vi "SetZControl.vi"(0 "Z Control Cluster":T1={"Input Signal"=0, "Min"=-inf, "Max"=-inf, "P"=-inf, "Setpoint a.u."=-inf, "Invert Polarity"=-2147483648, "I"=-inf} {"I" format="%#_g mHz"; "Invert Polarity" items=["[read only]"=-2147483648, "No"=0, "Yes"=1]; "Max" format="%#_g nm"; "Min" format="%#_g nm"; "Input Signal" items=["[read only]"=-2147483648, "ADC 1"=0, "ADC 2"=1, "ADC 3"=2, "ADC 4"=3, "ADC 5"=4, "ADC 6"=5, "HF 1 df"=8, "HF 1 Ampl"=13, "HF 1 Phase"=14, "LockIn Ampl"=16, "LockIn Phase"=17, "Counter"=23]}, 5 "error in":T4) -> (14 "Z Control Output":T1={"Input Signal"=0, "Min"=-inf, "Max"=-inf, "P"=-inf, "Setpoint a.u."=-inf, "Invert Polarity"=-2147483648, "I"=-inf} {"I" format="%#_g mHz"; "Invert Polarity" items=["[read only]"=-2147483648, "No"=0, "Yes"=1]; "Max" format="%#_g nm"; "Min" format="%#_g nm"; "Input Signal" items=["[read only]"=-2147483648, "ADC 1"=0, "ADC 2"=1, "ADC 3"=2, "ADC 4"=3, "ADC 5"=4, "ADC 6"=5, "HF 1 df"=8, "HF 1 Ampl"=13, "HF 1 Phase"=14, "LockIn Ampl"=16, "LockIn Phase"=17, "Counter"=23]}, 19 "error out":T4)   [LabVIEW 2016]
doc: "This VI prepares the z control by setting up all necessary parameters. Those are bundled in 'Z Control Cluster':\n\n- Actual Value (integer) [0-5 -- ADC1-6; 8 -- AFM df; 13 -- AFM Aosc; 14 -- AFM Phase; 16 -- LockIn Ampl; 17 -- LockIn Phase]\n- Min in nm (float) [0 to infinity]\n- Max in nm (float) [0 to infinity]\n- P (float) [0 to 100]\n- I in mHz (float) [without restraint]\n- Setpoint in mV, Hz or deg depending on the input \"Actual Value\". (float) [without restraint]\n- Invert Polarity (integer) [0 -- no; 1 -- yes]\n- Absolute (integer) [0 -- off; 1 -- on]\nBy passing -Inf (float) or -2147483648 (integer) as input values, the corresponding parameter(s) will be read out."
uses:
  Controls/Error_Out.ctl
  Controls/Z-Control_Parameters.ctl
  Controls/Actual-Value_Selection.ctl
  Controls/Invert-Polarity_Selection.ctl
  Files_ASC500/DLL/ASC500_RemoteControlV27.dll
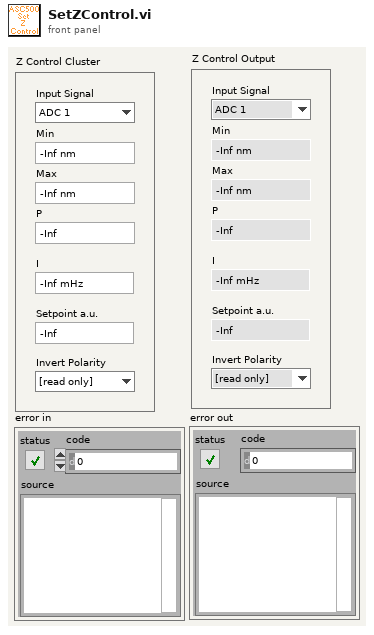
[diagram p1: front panel]
types:
  T1 = typedef "Z-Control_Parameters.ctl" = cluster{"Input Signal":T2, "Min":dbl, "Max":dbl, "P":dbl, "Setpoint a.u.":dbl, "Invert Polarity":T3, "I":dbl}
  T2 = typedef "Actual-Value_Selection.ctl" = i32
  T3 = typedef "Invert-Polarity_Selection.ctl" = i32
  T4 = typedef "Error_Out.ctl" = errorcluster
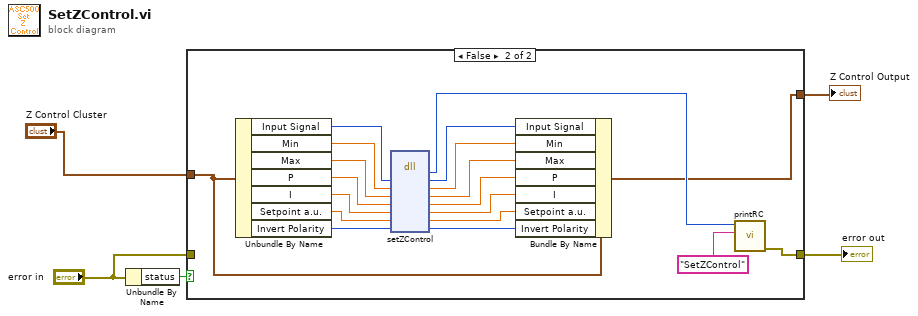
[diagram p0: block diagram]
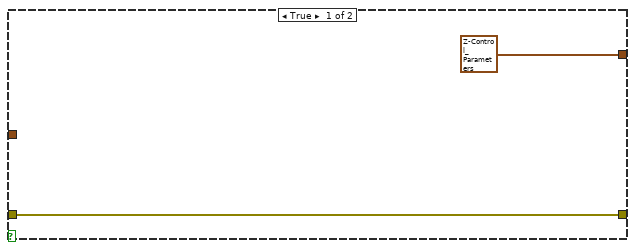
[diagram p2: hidden frame]
diagram:
  n1 = Unbundle By Name("error in") -> ("status"=w5:bool)
  n2 = case shown="False" w5 {
    tunnel: [w7 w10] -> w4
    tunnel: "error in" -> [w7 _]
    tunnel: "Z Control Cluster" -> [_ w9]
    tunnel: [T1 {"Input Signal"=0, "Min"=-inf, "Max"=-inf, "P"=-inf, "Setpoint a.u."=-inf, "Invert Polarity"=-2147483648, "I"=-inf} ("Z Control Cluster 2") w8] -> w1
    frame True {
    }
    frame False {
      n3 = Unbundle By Name(w9) -> ("Input Signal"=w26:T2, "Min"=w25:dbl, "Max"=w24:dbl, "P"=w23:dbl, "I"=w22:dbl, "Setpoint a.u."=w21:dbl, "Invert Polarity"=w20:T3)
      n4 = dll-call lib="G:/SCMOperations/Share/ELE/Produkt Information/ASC500/04 Remote Control/02 development versions/2018Nov06/Files_ASC500/DLL/ASC500_RemoteControlV27.dll" fn="setZControl"("Actual Value"=w26, "Min"=w25, "Max"=w24, "P"=w23, "I"=w22, "Setpoint"=w21, "Invert Polarity"=w20) -> ("return type"=w12:i32, "Actual Value"=w13:i32, "Min"=w14:sgl, "Max"=w15:sgl, "P"=w16:sgl, "I"=w17:sgl, "Setpoint"=w18:sgl, "Invert Polarity"=w19:i32)  [unwired: 3 in, 2 out]
      n5 = Bundle By Name(cluster=w9, "Input Signal"=w13, "Min"=w14, "Max"=w15, "P"=w16, "I"=w17, "Setpoint a.u."=w18, "Invert Polarity"=w19) -> (w8:T1)
      n6 = call "printRC.vi"("additional information"="SetZControl", "RC"=w12) -> ("error out"=w10:T4)  [unwired: 9 in]
    }
  }
  "error out" <- w4
  "Z Control Output" <- w1
